vi "Sub_square_from_csv.vi"(11 "To Flattened":dbl[][](array[numeric])) -> (3 "Square":dbl[][](array[numeric]))   [LabVIEW 2021]
panel:
  out "element":dbl
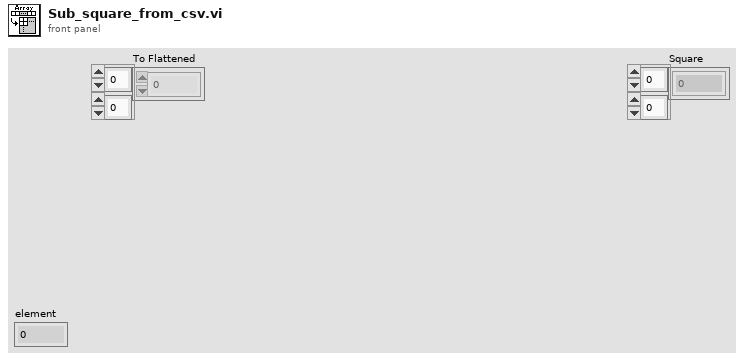
[diagram p1: front panel]
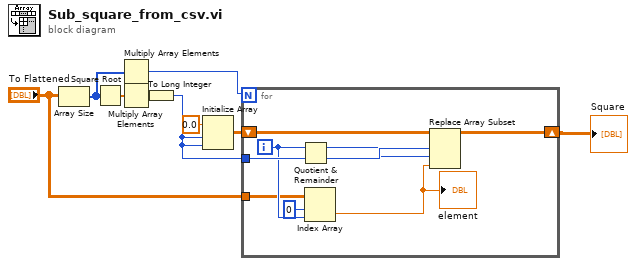
[diagram p0: block diagram]
diagram:
  n1 = Array Size(array="To Flattened") -> (size(s)=w4:i32[])
  n2 = Square Root(x=w4) -> (sqrt(x)=w9:dbl[])
  n3 = Multiply Array Elements(1:w4) -> (0:w3:i32)
  n4 = Multiply Array Elements(1:w9) -> (0:w8:dbl)
  n5 = To Long Integer(number=w8) -> (32bit integer=w2:i32)
  n6 = Initialize Array(0.0 ("element"), w2, w2) -> (w7:dbl[][])
  n7 = for {
    N: w3 -> [_]
    tunnel: "To Flattened" -> [w11]
    shift-right: [w18] -> w5
    shift-left: w7 -> [w12]
    tunnel: w2 -> [w15]
    i -> [w14]
    n8 = Quotient & Remainder(x=w14, y=w15) -> (x-y*floor(x/y)=w16:i32, floor(x/y)=w17:i32)
    n9 = Index Array(array=w11, index (row)=0 ("disabled index (row)"), index (col)=w14) -> (element=w13:dbl)
    "element" <- w13
    n10 = Replace Array Subset(array=w12, new element=w13, index (row)=w17, index (col)=w16) -> (w18:dbl[][])
  }
  "Square" <- w5
